vi "Save Image to File.vi"(8 "错误输入（无错误）":errorcluster, 9 "Image Format":refnum<k24>, 10 "Image Save Path":path, 11 "Image Ref In":refnum<k24>) -> (0 "错误输出":errorcluster, 3 "Image Ref Out":refnum<k24>)   [LabVIEW 2012, in "Image Converter.lvlib"]
uses:
  Image Converter.lvlib
  System.Drawing
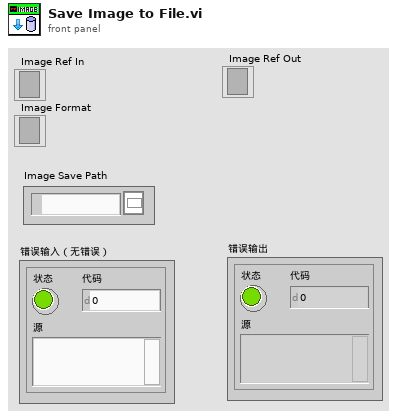
[diagram p1: front panel]
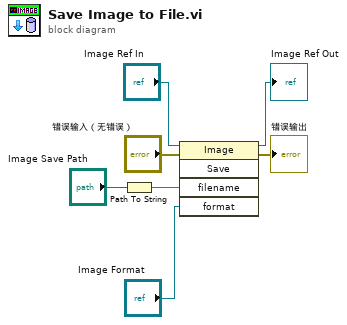
[diagram p0: block diagram]
diagram:
  n1 = Path To String(path="Image Save Path") -> (string=w1:string)
  n2 = invoke class="Image" method="Save"(reference="Image Ref In", error in="错误输入（无错误）", "filename"=w1, "format"="Image Format") -> (reference out=→"Image Ref Out":refnum<k24>, error out=→"错误输出":errorcluster)  [unwired: 1 in, 3 out]
